vi "Number Split.VI"(0 "number string":string, 1 "error in (no error)":errorcluster) -> (2 "number":string, 3 "rest":string, 4 "error out":errorcluster)   [LabVIEW 2024, in "NI_Gmath.lvlib"]
uses:
  NI_Gmath.lvlib
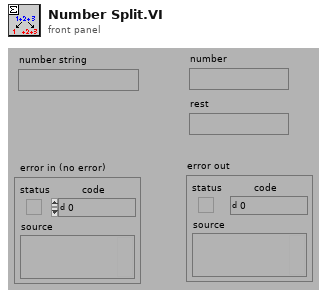
[diagram p1: front panel]
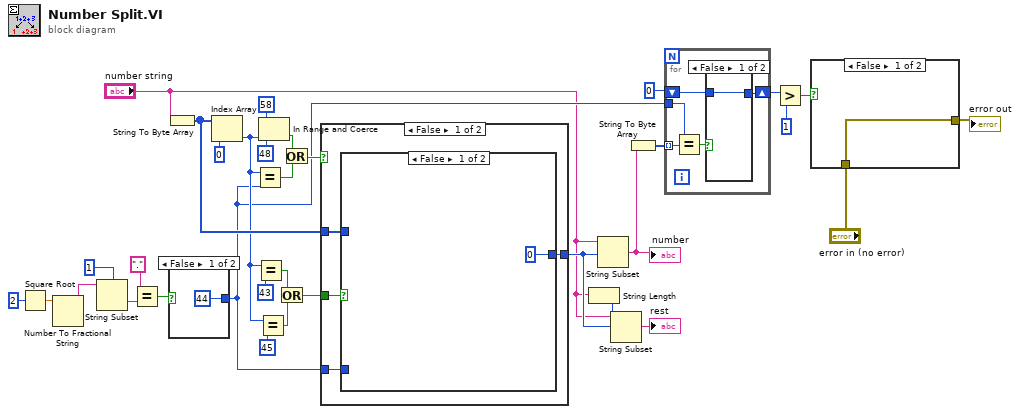
[diagram p0: block diagram]
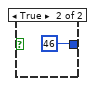
[diagram p2: hidden frame]
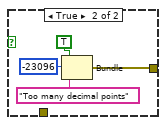
[diagram p3: hidden frame]
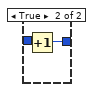
[diagram p4: hidden frame]
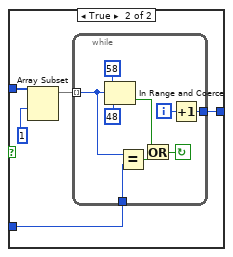
[diagram p5: hidden frame]
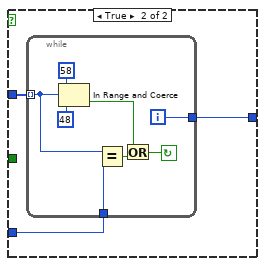
[diagram p6: hidden frame]
diagram:
  w10 = 1
  n1 = Square Root(x=2) -> (sqrt(x)=w8:dbl)
  n2 = Number To Fractional String(number=w8) -> (F-format string=w11:string)  [unwired: 3 in]
  n3 = String Subset(string=w11, offset (0)=w10, length (rest)=w10) -> (substring=w7:string)
  n4 = Equal?(x=".", y=w7) -> (x = y?=w5:bool)
  n5 = String To Byte Array(string="number string") -> (unsigned byte array=w30:u8[])
  n6 = case shown="False" w5 {
    tunnel: [44 46] -> w4
    frame False {
    }
    frame True {
    }
  }
  n7 = Index Array(array=w30, index=0) -> (element=w23:u8)
  n8 = Equal?(x=w23, y=w4) -> (x = y?=w25:bool)
  n9 = Equal?(x=w23, y=43) -> (x = y?=w20:bool)
  n10 = Equal?(x=w23, y=45) -> (x = y?=w19:bool)
  n11 = In Range and Coerce(upper limit=58, x=w23, lower limit=48) -> (In Range?=w26:bool)  [unwired: 1 out]
  n12 = Or(x=w20, y=w19) -> (x .or. y?=w18:bool)
  n13 = Or(x=w26, y=w25) -> (x .or. y?=w24:bool)
  n14 = case shown="False" w24 {
    tunnel: w30 -> [w38 w57]
    tunnel: [w37 w56] -> w27
    tunnel: w18 -> [w39 _]
    tunnel: w4 -> [w36 w55]
    frame False {
      n15 = case shown="False" w39 {
        tunnel: w38 -> [_ w43]
        tunnel: [0 w45] -> w37
        tunnel: w36 -> [_ w41]
        frame False {
        }
        frame True {
          n16 = Array Subset(array=w43, index=1) -> (w44:u8[])  [unwired: 1 in]
          n17 = while {
            tunnel: w41 -> [w46]
            tunnel: [w47] -> w45
            tunnel: w44 -> [w52] mode=indexing
            i -> [w48]
            stop <- w49 continue-if-true
            n18 = In Range and Coerce(upper limit=58, x=w52, lower limit=48) -> (In Range?=w50:bool)  [unwired: 1 out]
            n19 = Equal?(x=w52, y=w46) -> (x = y?=w51:bool)
            n20 = Or(x=w50, y=w51) -> (x .or. y?=w49:bool)
            n21 = Increment(x=w48) -> (x+1=w47:i32)
          }
        }
      }
    }
    frame True {
      n22 = while {
        tunnel: w55 -> [w58]
        tunnel: [w59] -> w56
        tunnel: w57 -> [w63] mode=indexing
        i -> [w59]
        stop <- w60 continue-if-true
        n23 = In Range and Coerce(upper limit=58, x=w63, lower limit=48) -> (In Range?=w61:bool)  [unwired: 1 out]
        n24 = Equal?(x=w63, y=w58) -> (x = y?=w62:bool)
        n25 = Or(x=w61, y=w62) -> (x .or. y?=w60:bool)
      }
    }
  }
  n26 = String Length(string="number string") -> (length=w29:i32)
  n27 = String Subset(string="number string", length (rest)=w27) -> (substring=w17:string)  [unwired: 1 in]
  "number" <- w17
  n28 = String Subset(string="number string", offset (0)=w27, length (rest)=w29) -> (substring=→"rest":string)
  n29 = String To Byte Array(string=w17) -> (unsigned byte array=w16:u8[])
  n30 = for {
    tunnel: w16 -> [w70] mode=indexing
    shift-right: [w67] -> w14
    shift-left: 0 -> [w68]
    tunnel: w4 -> [w66]
    n31 = Equal?(x=w66, y=w70) -> (x = y?=w69:bool)
    n32 = case shown="False" w69 {
      tunnel: w68 -> [w71 w73]
      tunnel: [w71 w72] -> w67
      frame False {
      }
      frame True {
        n33 = Increment(x=w73) -> (x+1=w72:i32)
      }
    }
  }
  n34 = Greater?(x=w14, y=1) -> (0:w12:bool)
  n35 = case shown="False" w12 {
    tunnel: "error in (no error)" -> [w74 _]
    tunnel: [w74 w77] -> w2
    frame False {
    }
    frame True {
      n36 = Bundle(TRUE, -23096, "number string"="Too many decimal points") -> (w77:cluster{bool, i32, "number string":string})  [unwired: 1 in]
    }
  }
  "error out" <- w2
